vi "PlayVideo.vi"(8 "error in (no error)":errorcluster, 11 "CameraTestingBL in":refnum<class "CameraTesting.lvclass">) -> (0 "error out":errorcluster, 3 "CameraTestingBL out":refnum<class "CameraTesting.lvclass">)   [LabVIEW 2020, in "CameraTesting.lvlib" / "CameraTesting.lvclass"]
doc: "Send command to camera to starting the data streaming"
uses:
  CameraTesting.lvclass
  CameraTesting.lvclass/CameraTesting.ctl
  Camera/ICamera/ICamera/ICamera.lvclass
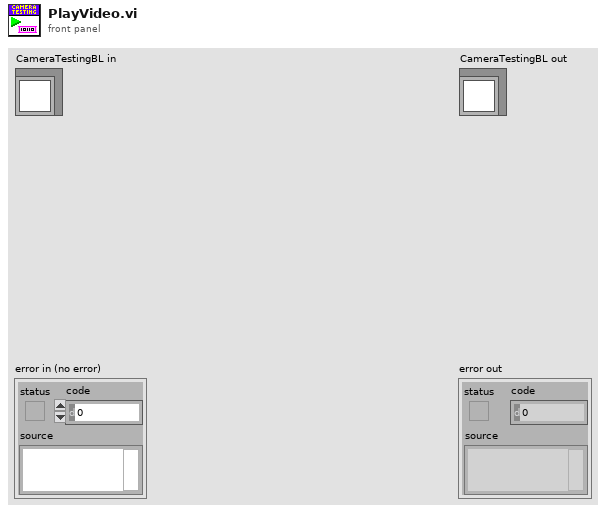
[diagram p1: front panel]
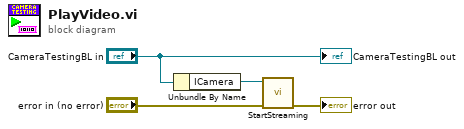
[diagram p0: block diagram]
diagram:
  n1 = Unbundle By Name("CameraTestingBL in") -> ("ICamera"=w4:refnum<class "ICamera.lvclass">)
  n2 = call-dynamic "StartStreaming.vi"("error in (no error)"="error in (no error)", "ICamera in"=w4) -> ("error out"=→"error out":errorcluster)  [unwired: 8 in, 1 out]
  "CameraTestingBL out" <- "CameraTestingBL in"
